vi "System Error Cluster Replacement.vi"(8 "error in (no error)":errorcluster, 11 "Folder Path":path) -> (0 "error out":errorcluster)   [LabVIEW 2020]
uses:
  <vilib>/Utility/traverseref.llb/TRef TravTarget.ctl
panel:
  out "Slide":i32(slide) caption="New Table.vi" scale=0.0..275.0
  out "VIs on Error":path[](array[path])
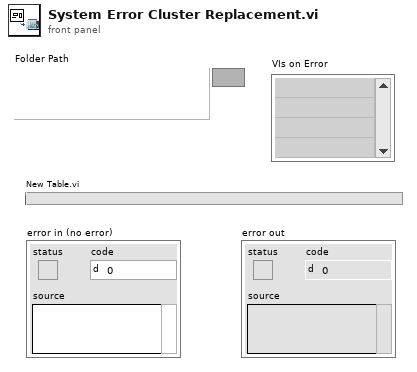
[diagram p1: front panel]
types:
  T1 = typedef "TRef TravTarget.ctl" = enum16{"FP", "BD", "Other"}
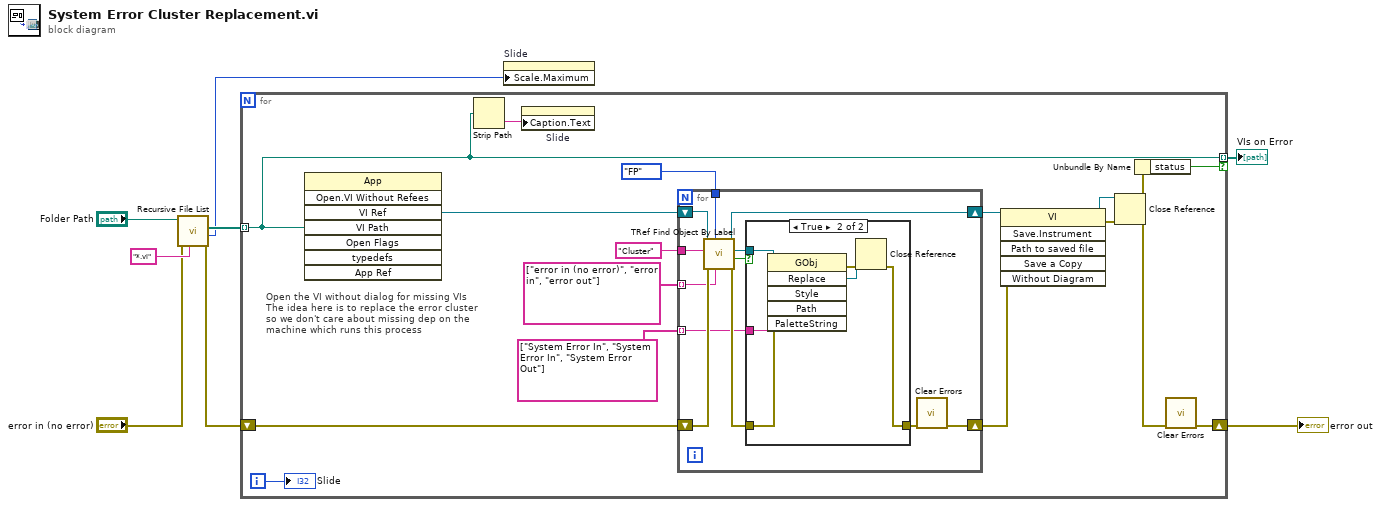
[diagram p0: block diagram]
diagram:
  n1 = call <vilib>:"Recursive File List.vi"("pattern"="*.vi", "error in (no error)"="error in (no error)", "Folder Path"="Folder Path") -> ("error out"=w3:errorcluster, "Number of Files"=w1:i32, "All Files in Dir"=w5:path[])  [unwired: 4 in, 2 out]
  n2 = for {
    shift-right: [w16] -> w8
    shift-left: w3 -> [w9]
    tunnel: w5 -> [w11] mode=indexing
    tunnel: [w11] -> w2 mode=indexing if=w14
    i -> [w13]
    # "Open the VI without dialog for missing VIs\nThe idea here is to replace the error cluster\nso we don't care about missing dep on the\nmachine which runs this process"
    n3 = invoke class="App" method="Open.VI Without Refees"("VI Path"=w11) -> ("VI Ref"=w10:refnum<vi>)  [unwired: 7 in, 7 out]
    n4 = Strip Path(path=w11) -> (name=w12:string)  [unwired: 1 out]
    n5 = property on="Slide" class="Slide (strict)"("Caption.Text"=w12) -> ()  [unwired: 2 in, 2 out]
    n6 = for {
      tunnel: TRef_TravTarget."FP" ("Traverse Target") -> [w35]
      tunnel: "Cluster" ("Class Name") -> [w34]
      shift-right: [w31] -> w20
      shift-left: w10 -> [w36]
      tunnel: string[] ["error in (no error)", "error in", "error out"] -> [w27] mode=indexing
      tunnel: string[] ["System Error In", "System Error In", "System Error Out"] -> [w26] mode=indexing
      shift-right: [w25] -> w19
      shift-left: w9 -> [w28]
      n7 = call <vilib>:"TRef Find Object By Label.vi"("Label"=w27, "Traverse Target"=w35, "error in (no error)"=w28, "Class Name"=w34, "VI Ref"=w36) -> ("error out"=w32:errorcluster, "Found?"=w29:bool, "Found Obj Ref"=w33:refnum<vi>, "dup VI Ref"=w31:refnum<vi>)  [unwired: 3 in]
      n8 = case shown="True" w29 {
        tunnel: w33 -> [_ w43]
        tunnel: w32 -> [w37 w42]
        tunnel: w26 -> [_ w41]
        tunnel: [w37 w39] -> w30
        frame False {
        }
        frame True {
          n9 = invoke class="GObj" method="Replace"(reference=w43, error in=w42, "PaletteString"=w41) -> (error out=w40:errorcluster, "Replace"=w38:refnum<vi>)  [unwired: 3 in, 4 out]
          n10 = Close Reference(reference=w38, error in (no error)=w40) -> (error out=w39:errorcluster)
        }
      }
      n11 = call <vilib>:"Clear Errors.vi"("error in (no error)"=w30) -> ("error out"=w25:errorcluster)  [unwired: 5 in, 1 out]
    }
    n12 = invoke class="VI" method="Save.Instrument"(reference=w20, error in=w19) -> (reference out=w18:refnum<vi>, error out=w17:errorcluster)  [unwired: 4 in, 4 out]
    n13 = Close Reference(reference=w18, error in (no error)=w17) -> (error out=w15:errorcluster)
    n14 = Unbundle By Name(w15) -> ("status"=w14:bool)
    n15 = call <vilib>:"Clear Errors.vi"("error in (no error)"=w15) -> ("error out"=w16:errorcluster)  [unwired: 5 in, 1 out]
    "Slide" <- w13
  }
  "error out" <- w8
  "VIs on Error" <- w2
  n16 = property on="Slide" class="Slide (strict)"("Scale.Maximum"=w1) -> ()  [unwired: 2 in, 2 out]
